vi "Launch New Chat Window.vi"(8 "error in (no error)":errorcluster, 11 "Server in":refnum<class "Server.lvclass">) -> (0 "error out":errorcluster, 3 "Server out":refnum<class "Server.lvclass">)   [LabVIEW 2019, in "Server.lvlib" / "Server.lvclass"]
uses:
  Server.lvclass
  C:/Program Files (x86)/National Instruments/LabVIEW 2019/vi.lib/ActorFramework/Actor/Actor.lvclass
  Chat Room Model/Chat Room Model/Chat Room Model.lvclass
  Server.lvclass/Server.ctl
  <vilib>/ActorFramework/Actor/Actor.lvclass
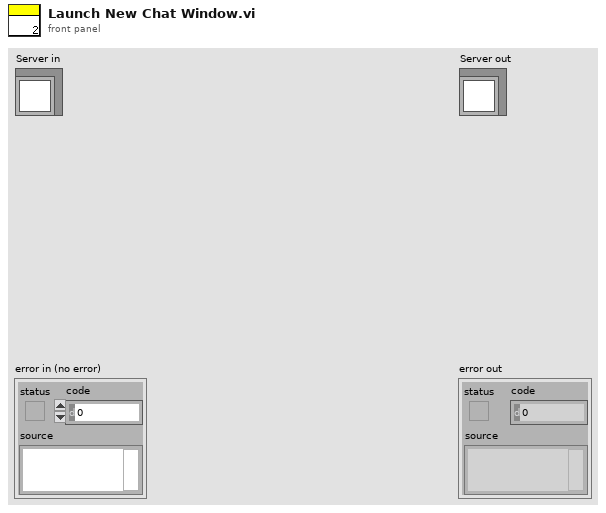
[diagram p1: front panel]
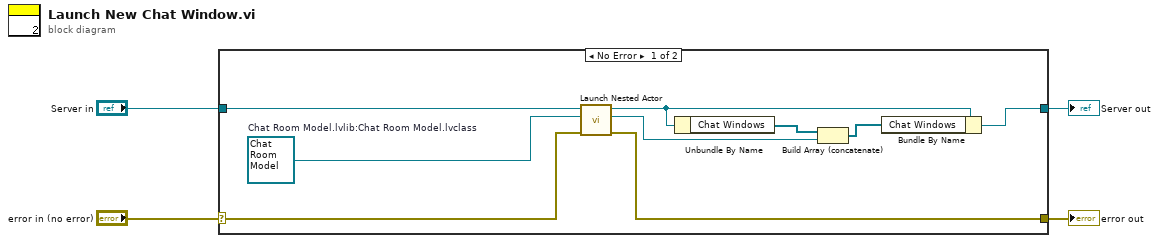
[diagram p0: block diagram]
diagram:
  n1 = case shown="No Error" "error in (no error)" {
    selector: "error in (no error)" -> [w13 w15]
    tunnel: [w12 w15] -> w3
    tunnel: [w9 w14] -> w1
    tunnel: "Server in" -> [w11 w14]
    frame No Error {
      w10 = refnum<class "Chat Room Model.lvclass"> refnum  # Chat Room Model.lvlib:Chat Room Model.lvclass
      n2 = call <vilib>:"Launch Nested Actor.vi"("error in (no error)"=w13, "Nested Actor"=w10, "Caller Actor in"=w11) -> ("error out"=w12:errorcluster, "Nested Actor's Enqueuer"=w6:refnum<class "Message Enqueuer.lvclass">, "Caller Actor out"=w8:refnum<class "Server.lvclass">)  [unwired: 6 in]
      n3 = Unbundle By Name(w8) -> ("Chat Windows"=w7:refnum<class "Message Enqueuer.lvclass">[])
      n4 = Build Array (concatenate)(w7, w6) -> (w5:refnum<class "Message Enqueuer.lvclass">[])
      n5 = Bundle By Name(cluster=w8, "Chat Windows"=w5) -> (w9:refnum<class "Server.lvclass">)
    }
    frame Error {
    }
  }
  "error out" <- w3
  "Server out" <- w1
